vi "Client Get Version on Server.vi"(8 "error in (no error)":errorcluster) -> (0 "error out":errorcluster, 2 "Version":T1 {"Build Date/Time" format="%<%X\n%x>T"}, 3 "Client EXE Name":string)   [LabVIEW 2011]
uses:
  Summitek EXT/Miscellaneous/OGAB Version.ctl
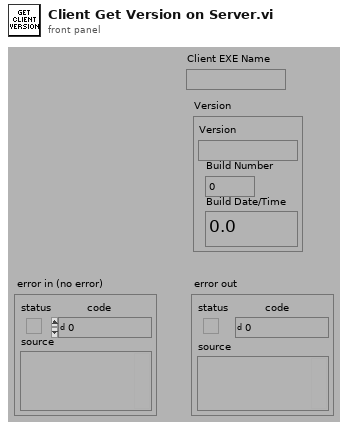
[diagram p1: front panel]
types:
  T1 = typedef "OGAB Version.ctl" = cluster{"Version":string, "Build Number":u32, "Build Date/Time":dbl}
  T2 = enum32{"invalid app kind", "Development System", "Run Time System", "Student Edition", "Embedded LabVIEW", "Evaluation", "Custom"}
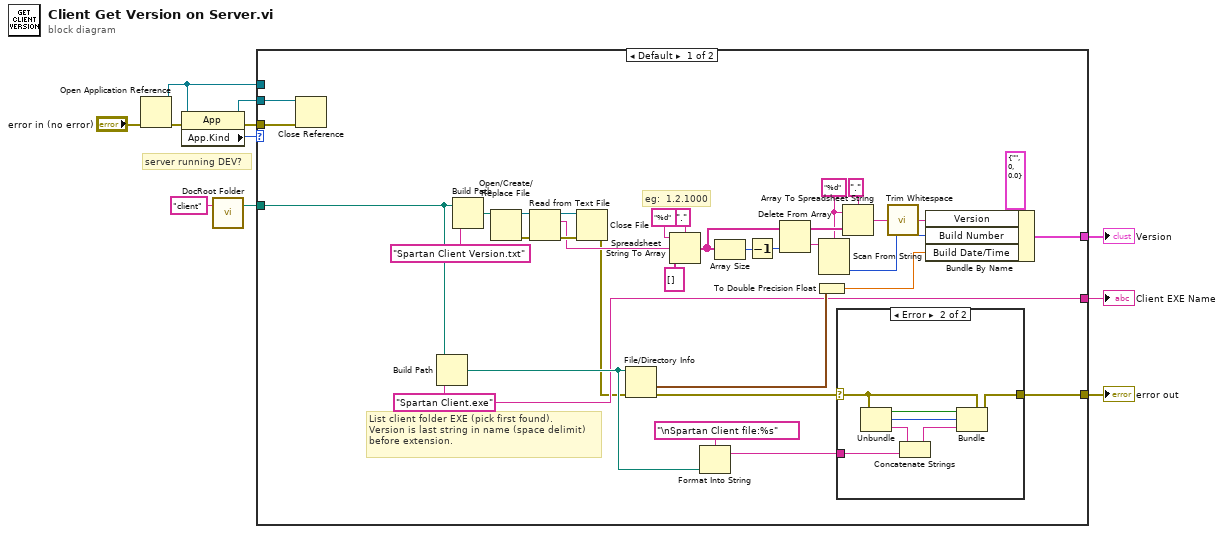
[diagram p0: block diagram]
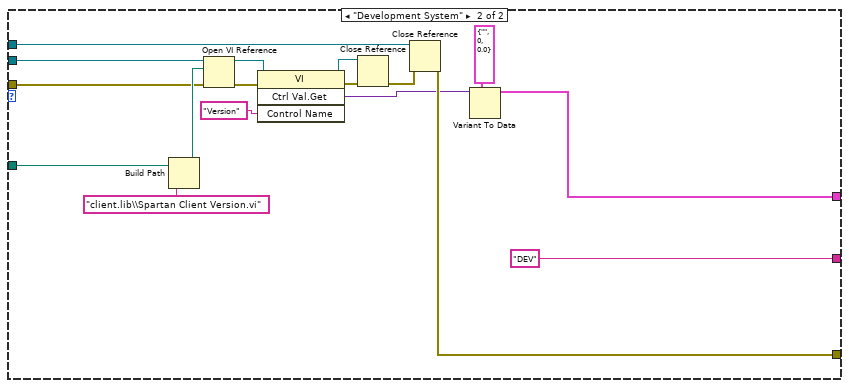
[diagram p3: hidden frame]
diagram:
  # "server running DEV?"
  n1 = Open Application Reference(8:"error in (no error)") -> (0:w5:errorcluster, 3:w4:refnum<vi>)  [unwired: 3 in]
  n2 = property class="App"(reference=w4, error in=w5) -> (reference out=w8:refnum<vi>, error out=w7:errorcluster, "App.Kind"=w1:T2)
  n3 = call "DocRoot Folder.vi"("Relative Path (\"\" - Folder)"="client" ("stripped path")) -> ("DocumentRoot Folder"=w2:path)  [unwired: 2 in]
  n4 = case shown="Default" w1 {
    tunnel: [w45 w54] -> w11
    tunnel: [w13 "DEV"] -> w10
    tunnel: [w44 w58] -> w9
    tunnel: w2 -> [w21 w70]
    tunnel: w8 -> [w24 w68]
    tunnel: w7 -> [w23 w66]
    tunnel: w4 -> [_ w62]
    frame Default {
      w13 = "Spartan Client.exe" ("name or relative path")
      w30 = "%d" ("format string")
      # "eg:  1.2.1000"
      # "List client folder EXE (pick first found).\nVersion is last string in name (space delimit)\nbefore extension."
      n5 = Close Reference(reference=w24, error in (no error)=w23) -> ()  [unwired: 1 out]
      n6 = Build Path(base path=w21, name or relative path=w13) -> (appended path=w14:path)
      n7 = Build Path(base path=w21, name or relative path="Spartan Client Version.txt") -> (appended path=w16:path)
      n8 = Open/Create/Replace File(file path (use dialog)=w16) -> (refnum out=w20:refnum<file>, error out=w17:errorcluster)  [unwired: 5 in, 1 out]
      n9 = Read from Text File(file (use dialog)=w20, error in=w17) -> (refnum out=w19:refnum<file>, text=w15:string, error out=w18:errorcluster)  [unwired: 2 in, 1 out]
      n10 = Close File(refnum=w19, error in=w18) -> (error out=w12:errorcluster)  [unwired: 1 out]
      n11 = File/Directory Info(path=w14, error in=w12) -> (last mod=w42:timestamp, error out=w26:errorcluster)  [unwired: 5 out]
      n12 = Spreadsheet String To Array(delimiter (Tab)=".", format string="%d", spreadsheet string=w15, array type (2D Dbl)=string[] []) -> (array=w37:string[])
      n13 = Format Into String(format string="\nSpartan Client file:%s", w14) -> (resulting string=w25:string)  [unwired: 2 in, 1 out]
      n14 = Array Size(array=w37) -> (size(s)=w36:i32)
      n15 = Decrement(x=w36) -> (x-1=w35:i32)
      n16 = Delete From Array(array=w37, index=w35) -> (deleted portion=w32:string, array with subset deleted=w34:string[])  [unwired: 1 in]
      n17 = To Double Precision Float(number=w42) -> (double precision float=w41:dbl)
      n18 = Scan From String(format string=w30, input string=w32) -> (output 1=w31:i32)  [unwired: 2 in, 4 out]
      n19 = case shown="Error" w26 {
        selector: w26 -> [w46 w52]
        tunnel: [w46 w49] -> w44
        tunnel: w25 -> [_ w48]
        frame No Error {
        }
        frame Error {
          n20 = Unbundle(w52) -> ("status"=w51:bool, "code"=w50:i32, "source"=w53:string)
          n21 = Concatenate Strings(w53, w48) -> (w47:string)
          n22 = Bundle(cluster=w52, "status"=w51, "code"=w50, "source"=w47) -> (w49:errorcluster)
        }
      }
      n23 = Array To Spreadsheet String(delimiter (Tab)=".", array=w34, 3:w30) -> (spreadsheet string=w29:string)
      n24 = call <vilib>:"Trim Whitespace.vi"("string"=w29) -> ("trimmed string"=w28:string)  [unwired: 1 in]
      n25 = Bundle By Name(cluster=T1 {"Version"="", "Build Number"=0, "Build Date/Time"=0.0} ("Version"), "Version"=w28, "Build Number"=w31, "Build Date/Time"=w41) -> (w45:T1)
    }
    frame "Development System" {
      n26 = Build Path(base path=w70, name or relative path="client.lib\\Spartan Client Version.vi") -> (appended path=w67:path)
      n27 = Open VI Reference(application reference (local)=w68, vi path=w67, error in (no error)=w66) -> (vi reference=w64:refnum<vi>, error out=w65:errorcluster)  [unwired: 3 in]
      n28 = invoke class="VI" method="Ctrl Val.Get"(reference=w64, error in=w65, "Control Name"="Version" ("name or relative path")) -> (reference out=w59:refnum<vi>, error out=w60:errorcluster, "Get Control Value Variant"=w56:variant)  [unwired: 1 in, 1 out]
      n29 = Close Reference(reference=w59, error in (no error)=w60) -> (error out=w61:errorcluster)
      n30 = Close Reference(reference=w62, error in (no error)=w61) -> (error out=w58:errorcluster)
      n31 = Variant To Data(type=T1 {"Version"="", "Build Number"=0, "Build Date/Time"=0.0} ("Version"), Variant=w56) -> (data=w54:T1)  [unwired: 1 in, 1 out]
    }
  }
  "error out" <- w9
  "Version" <- w11
  "Client EXE Name" <- w10
